vi "624WPI_CameraSend Images To PC Loop.vi"(4 "error in (no error) 2":errorcluster, 6 "port 2":u16=1180, 8 "CameraDevRef 2":T1, 9 "error in (no error)":errorcluster, 10 "port":u16=1180, 11 "CameraDevRef":T1) -> ()   [LabVIEW 2014]
doc: "This VI is used to send images to the dashboard using the second enet port on the 8 slot controller. This is provided for compatibility, but is higher overhead than using the Camera MJPG approach.\n\nThis software is licensed. Open the labview\\readme\\WPI Robotics Library Open Source License.txt file for more information."
uses:
  <vilib>/Rock Robotics/WPI/Camera/WPI_CameraDevRef.ctl
  <vilib>/Rock Robotics/SystemInterfaces/NetworkCommunication/NetComm_UsageReport_ResourceType.ctl
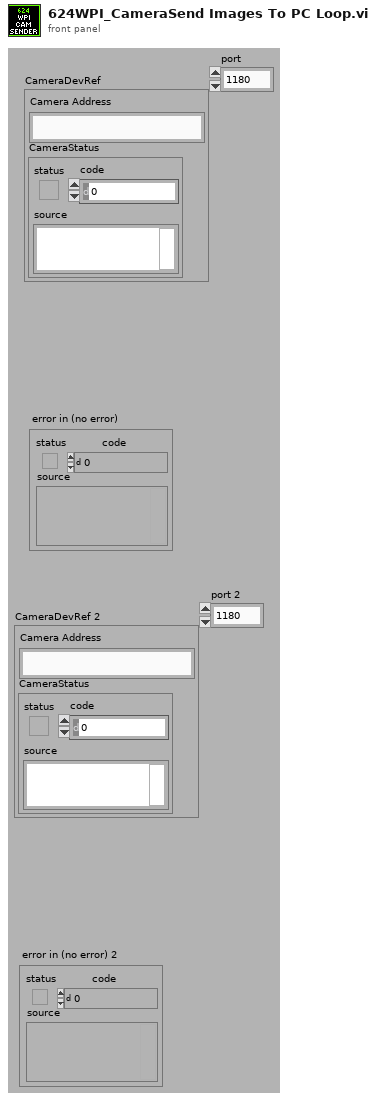
[diagram p1: front panel]
types:
  T1 = typedef "WPI_CameraDevRef.ctl" = cluster{"Camera Address":string, "CameraStatus":errorcluster}
  T2 = cluster{"fps":i32, "compression":i32, "compression 2":i32}
  T3 = typedef "NetComm_UsageReport_ResourceType.ctl" = enum8{"Controller", "Module", "Language", "CANPlugin", "Accelerometer", "ADXL345", "AnalogChannel", "AnalogTrigger", "AnalogTriggerOutput", "CANJaguar", "Compressor", "Counter", "Dashboard", "DigitalInput", "DigitalOutput", "DriverStationCIO", "DriverStationEIO", "DriverStationLCD", "Encoder", "GearTooth", "Gyro", "I2C", "Framework", "Jaguar", "Joystick", "Kinect", "KinectStick", "PIDController", "Preferences", "PWM", "Relay", "RobotDrive", "SerialPort", "Servo", "Solenoid", "SPI", "Task", "Ultrasonic", "Victor", "Button", "Command", "AxisCamera", "PCVideoServer", "SmartDashboard", "Talon", "HiTechnicColorSensor", "HiTechnicAccel", "HiTechnicCompass", "SRF08", "AnalogOutput", "Victor SP", "Talon SRX", "CAN Talon SRX"}
  T4 = enum16{"Update Mode", "Get Image", "Get Image Data"}
  T5 = typedef "Image Type" = u32
  T6 = typedef "IMAQ Image.ctl" = refnum<image>
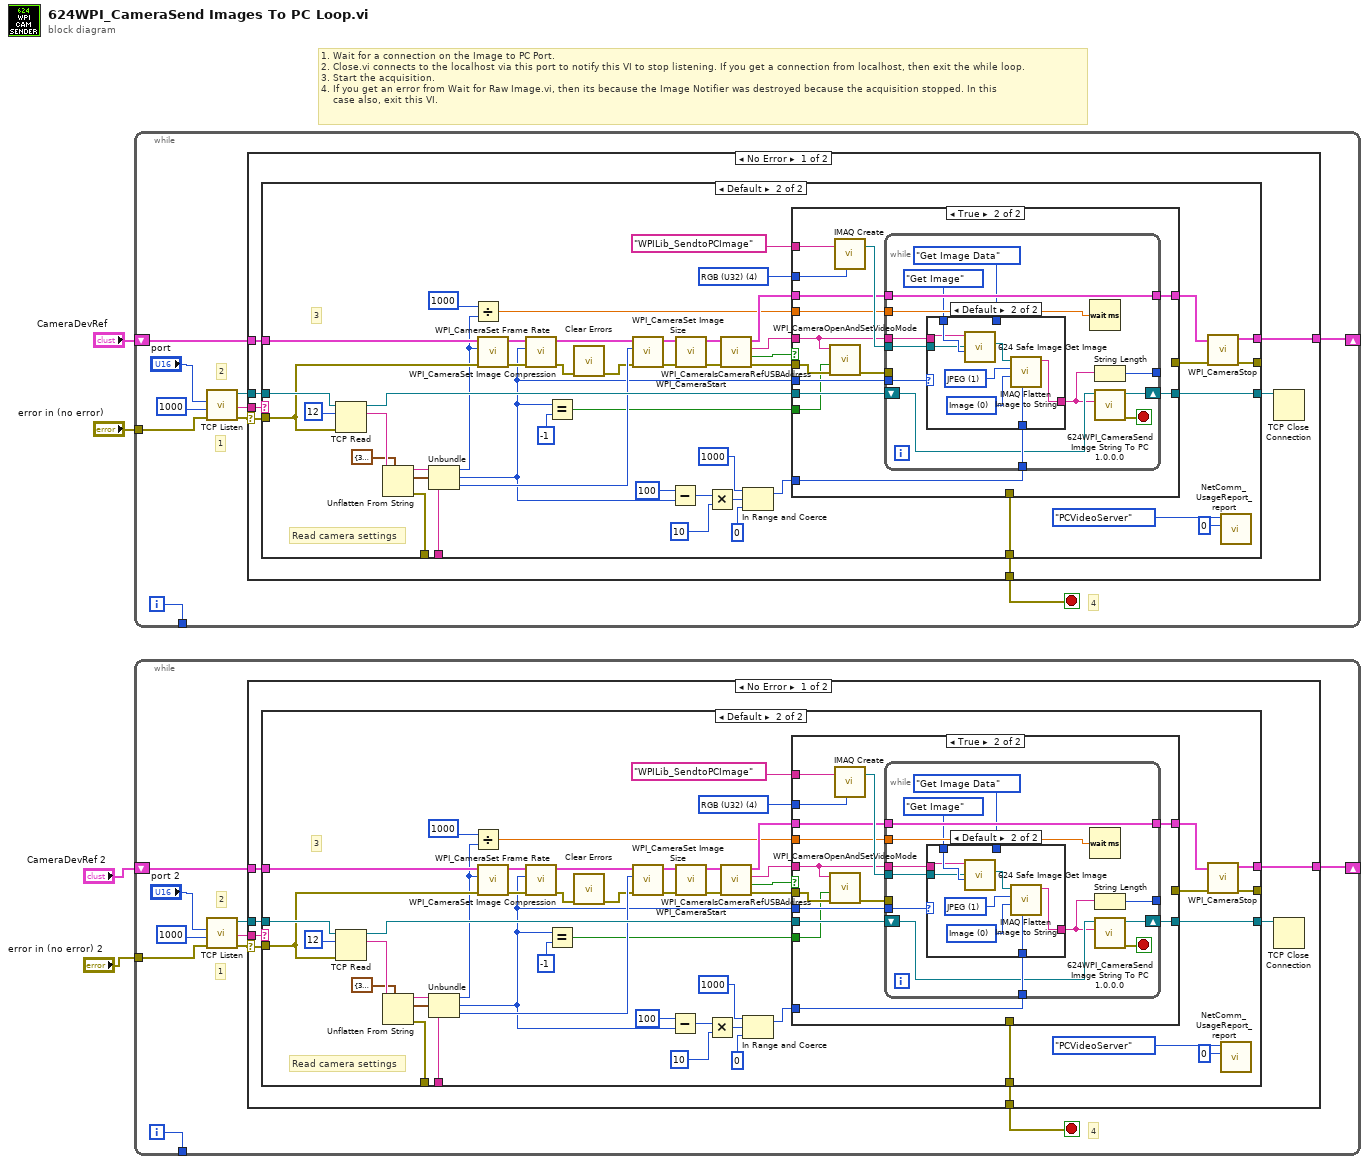
[diagram p0: block diagram]
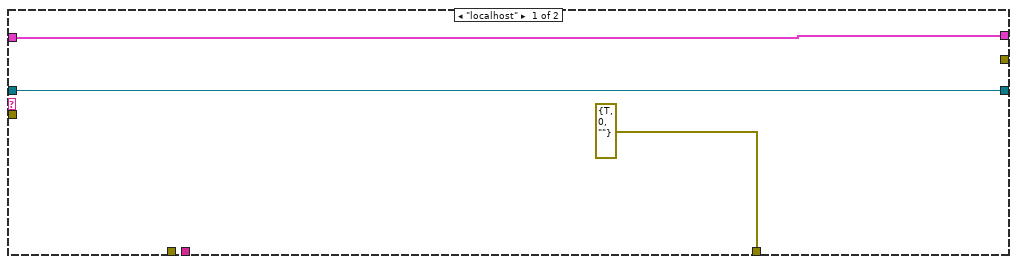
[diagram p2: hidden frame]
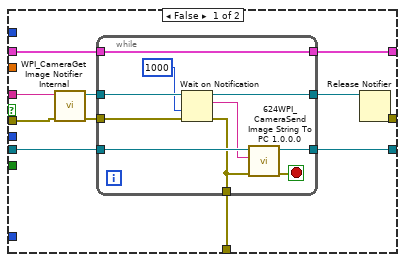
[diagram p3: hidden frame]
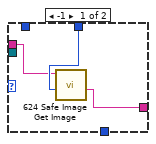
[diagram p4: hidden frame]
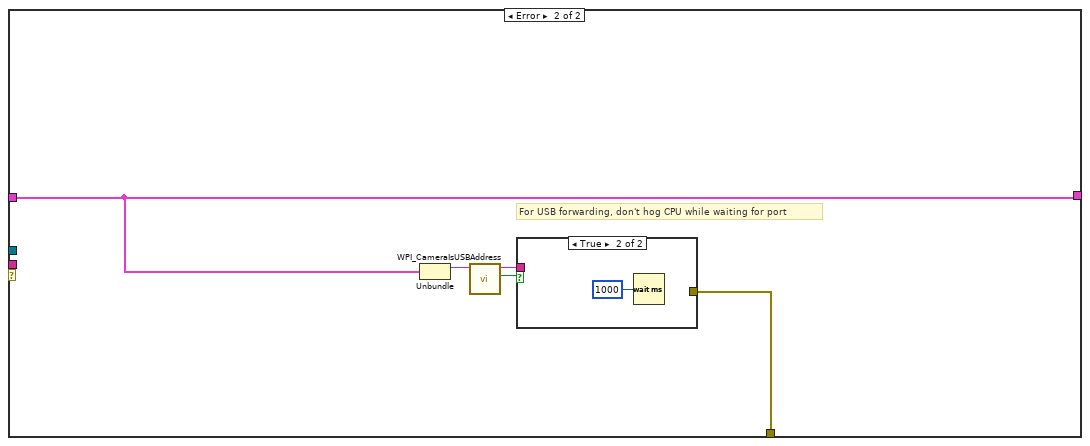
[diagram p5: hidden frame]
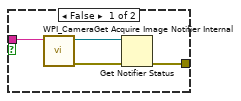
[diagram p6: hidden frame]
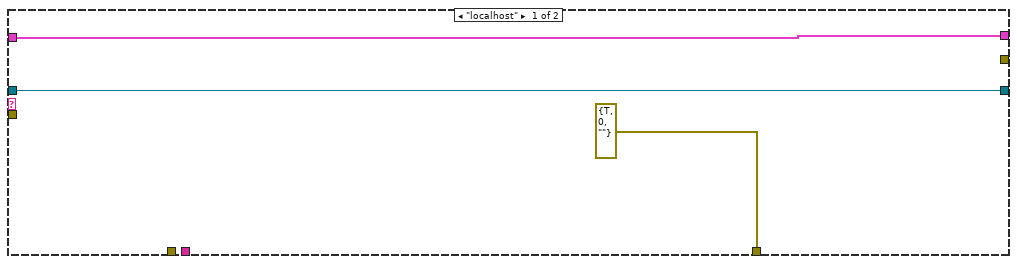
[diagram p7: hidden frame]
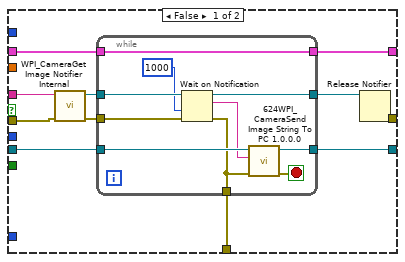
[diagram p8: hidden frame]
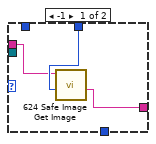
[diagram p9: hidden frame]
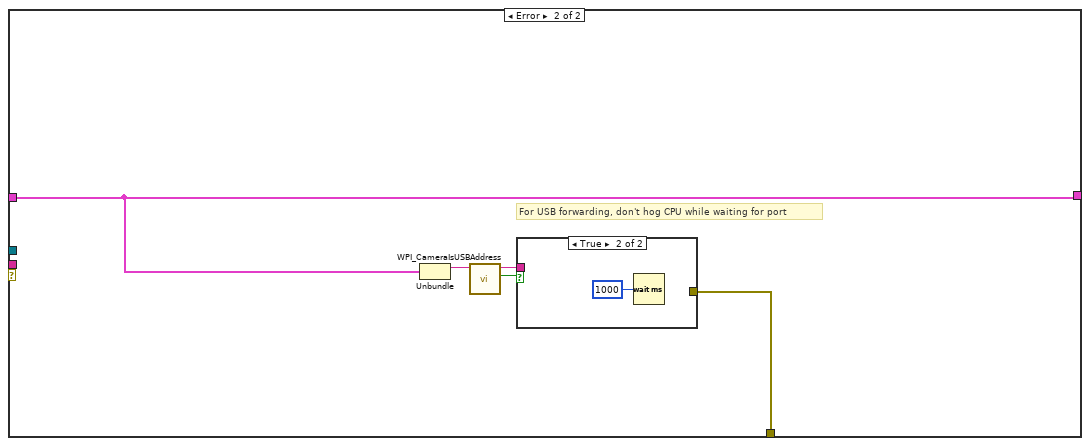
[diagram p10: hidden frame]
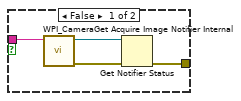
[diagram p11: hidden frame]
diagram:
  # "1. Wait for a connection on the Image to PC Port.\n2. Close.vi connects to the localhost via this port to notify this VI to stop listening. If you get a connection from localhost, then exit the while loop.\n3. Start the acquisition.\n4. If you get an error from Wait for Raw Image.vi, then its because the Image Notifier was destroyed because the acquisition stopped. In this\n    case also, exit this VI."
  n1 = while {
    tunnel: "error in (no error)" -> [w11]
    shift-right: [w14] -> _
    shift-left: "CameraDevRef" -> [w12]
    tunnel: [w6] -> _
    i -> [w6]
    stop <- w9 stop-if-true
    # "4"
    # "1"
    # "2"
    n2 = call <vilib>:"TCP Listen.vi"("error in (no error)"=w11, "timeout ms (wait forever: -1)"=u16 1000 ("port"), "port"="port") -> ("error out"=w8:errorcluster, "remote address"=w13:string, "connection ID"=w10:refnum<k5>)  [unwired: 1 in, 5 out]
    n3 = case shown="No Error" w8 {
      selector: w8 -> [w15 _]
      tunnel: [w21 w134] -> w14
      tunnel: w13 -> [w20 _]
      tunnel: w12 -> [w19 w134]
      tunnel: w10 -> [w18 _]
      tunnel: [w17 w135] -> w9
      frame No Error {
        n4 = case shown="Default" w20 {
          tunnel: [w24 w69] -> w21
          tunnel: w19 -> [w24 w51]
          tunnel: w15 -> [_ w47]
          tunnel: w18 -> [w22 w55]
          tunnel: [errorcluster {"status"=TRUE, "code"=0, "source"=""} ("error out 2") w71] -> w17
          tunnel: [w22 w70] -> w16
          tunnel: [_ w68] -> _
          tunnel: [_ w26] -> _
          tunnel: [_ w25] -> _
          frame "localhost" {
          }
          frame Default {
            w62 = T5 4 items=["Grayscale (U8)", "Grayscale (I16)", "Grayscale (SGL)", "Complex (CSG)", "RGB (U32)", "HSL (U32)", "RGB (U64)", "Grayscale (U16)"] ("Image Type")
            # "Read camera settings"
            # "3"
            n5 = TCP Read(connection ID=w55, bytes to read=12, error in (no error)=w47) -> (connection ID out=w54:refnum<k5>, data out=w52:string)  [unwired: 2 in, 1 out]
            n6 = Unflatten From String(type=T2 {"fps"=30, "compression"=32, "compression 2"=32} ("Camera Settings"), binary string=w52) -> (rest of the binary string=w25:string, value=w44:T2, error out=w26:errorcluster)  [unwired: 3 in]
            n7 = Unbundle(w44) -> ("fps"=w41:i32, "compression"=w30:i32, "compression 2"=w43:i32)
            n8 = Divide(x=u16 1000 ("port"), y=w41) -> (x/y=w40:dbl)
            n9 = call <vilib>:"WPI_CameraSet Frame Rate.vi"("error in (no error)"=w47, "Frame Rate (fps)"=w41, "CameraDevRef"=w51) -> ("error out"=w46:errorcluster, "CameraDevRef Out"=w50:T1)  [unwired: 7 in]
            n10 = call <vilib>:"WPI_CameraSet Image Compression.vi"("error in (no error)"=w46, "Compression"=w30, "CameraDevRef"=w50) -> ("error out"=w28:errorcluster, "CameraDevRef Out"=w49:T1)  [unwired: 7 in]
            n11 = Equal?(x=w30, y=-1) -> (x = y?=w29:bool)
            n12 = call <vilib>:"Clear Errors.vi"("error in (no error)"=w28) -> ("error out"=w27:errorcluster)  [unwired: 5 in, 1 out]
            n13 = call <vilib>:"WPI_CameraSet Image Size.vi"("error in (no error)"=w27, "Image Size"=w43, "CameraDevRef"=w49) -> ("error out"=w45:errorcluster, "CameraDevRef Out"=w48:T1)  [unwired: 7 in]
            n14 = Subtract(x=100, y=w30) -> (x-y=w35:i32)
            n15 = call <vilib>:"WPI_CameraStart.vi"("error in (no error)"=w45, "CameraDevRef"=w48) -> ("error out"=w59:errorcluster, "CameraDevRef Out"=w57:T1)  [unwired: 8 out]
            n16 = Multiply(x=w35, y=10) -> (x*y=w37:i32)
            n17 = call <vilib>:"WPI_CameraIsCameraRefUSBAddress.vi"("error in (no error)"=w59, "CameraDevRef"=w57) -> ("error out"=w58:errorcluster, "USB?"=w60:bool, "Camera Address Out"=w61:string, "CameraDevRef out"=w56:T1)  [unwired: 6 in]
            n18 = In Range and Coerce(upper limit=1000, x=w37, lower limit=0) -> (coerced(x)=w33:i32)  [unwired: 1 out]
            n19 = case shown="True" w60 {
              tunnel: w54 -> [w82 w106]
              tunnel: [w81 _] -> w71
              tunnel: [w80 w105] -> w70
              tunnel: w58 -> [w79 w96]
              tunnel: w61 -> [w77 w95]
              tunnel: [w76 w100] -> w67
              tunnel: w56 -> [w75 w101]
              tunnel: [w73 _] -> w66
              tunnel: "WPILib_SendtoPCImage" -> [_ w103]
              tunnel: w62 -> [_ w102]
              tunnel: w33 -> [_ w99]
              tunnel: w40 -> [_ w98]
              tunnel: w30 -> [_ w97]
              tunnel: w29 -> [_ w93]
              frame False {
                n20 = call <vilib>:"WPI_CameraGet Image Notifier Internal.vi"("error in (no error)"=w79, "Camera Address"=w77) -> ("error out"=w78:errorcluster, "Image Notifier"=w74:refnum<notifier>)  [unwired: 8 out]
                n21 = while {
                  tunnel: w78 -> [w88]
                  tunnel: w82 -> [w92]
                  tunnel: [w85] -> w81
                  tunnel: [w90] -> w80
                  tunnel: [w89] -> w76
                  tunnel: w75 -> [w89]
                  tunnel: w74 -> [w87]
                  tunnel: [w83] -> w72
                  stop <- w91 stop-if-true
                  n22 = Wait on Notification(notifier=w87, timeout in ms (-1)=1000 ("Timeout in ms (-1)"), error in (no error)=w88) -> (notifier out=w83:refnum<notifier>, notification=w86:string, error out=w85:errorcluster)  [unwired: 2 out]
                  n23 = call "624WPI_CameraSend Image String To PC 1.0.0.0.vi"("error in (no error)"=w85, "String"=w86, "TCP Connection ID"=w92) -> ("error out"=w91:errorcluster, "TCP Connection ID out"=w90:refnum<k5>)  [unwired: 7 out]
                }
                n24 = Release Notifier(notifier=w72) -> (error out=w73:errorcluster)  [unwired: 1 in, 3 out]
              }
              frame True {
                n25 = call <vilib>:"WPI_CameraOpenAndSetVideoMode.vi"("error in (no error)"=w96, "USB JPEG"=w93, "Camera Address Out"=w95) -> ("error out"=w94:errorcluster)  [unwired: 8 in]
                n26 = call "IMAQ Create"("Image Name"=w103, "Image Type"=w102) -> ("New Image"=w104:T6)  [unwired: 3 in, 1 out]
                n27 = while {
                  tunnel: w95 -> [w118]
                  shift-right: [w119] -> w105
                  shift-left: w106 -> [w112]
                  tunnel: w104 -> [w117]
                  tunnel: [w115] -> w100
                  tunnel: w101 -> [w115]
                  tunnel: w99 -> [w114]
                  tunnel: w98 -> [w113]
                  tunnel: [w110] -> _
                  tunnel: w97 -> [w109]
                  tunnel: w94 -> [_]
                  stop <- w116 stop-if-true
                  n28 = case shown="Default" w109 {
                    tunnel: [w121 w130] -> w111
                    tunnel: w118 -> [w120 w125]
                    tunnel: w117 -> [_ w124]
                    tunnel: w114 -> [_ w127]
                    tunnel: T4."Get Image Data" ("Operation") -> [w122 _]
                    tunnel: T4."Get Image" ("Operation") -> [_ w126]
                    frame -1 {
                      n29 = call "624 Safe Image Get Image.vi"("Operation"=w122, "Session In"=w120) -> ("Image Data String"=w121:string)  [unwired: 6 in, 3 out]
                    }
                    frame Default {
                      w128 = 0 items=["Image", "Image and Vision Info", "Reference to Image"] ("Type of Flatten (Image and Vision Info)")
                      w129 = 1 items=["None", "JPEG", "PACKED BINARY"] ("Compression (None)")
                      n30 = call "624 Safe Image Get Image.vi"("Operation"=w126, "Image In"=w124, "Session In"=w125) -> ("Image Out"=w123:T6)  [unwired: 5 in, 3 out]
                      n31 = call "IMAQ Flatten Image to String"("Quality (750)"=w127, "Type of Flatten (Image and Vision Info)"=w128, "Compression (None)"=w129, "Image"=w123) -> ("Data String"=w130:string)  [unwired: 6 in, 1 out]
                    }
                  }
                  n32 = Wait (ms)(milliseconds to wait=w113) -> ()  [unwired: 1 out]
                  n33 = String Length(string=w111) -> (length=w110:i32)
                  n34 = call "624WPI_CameraSend Image String To PC 1.0.0.0.vi"("String"=w111, "TCP Connection ID"=w112) -> ("error out"=w116:errorcluster, "TCP Connection ID out"=w119:refnum<k5>)  [unwired: 1 in, 7 out]
                }
              }
            }
            n35 = call <vilib>:"WPI_CameraStop.vi"("error in (no error)"=w66, "CameraDevRef"=w67) -> ("error out"=w68:errorcluster, "CameraDevRef Out"=w69:T1)  [unwired: 8 out]
            n36 = call <vilib>:"NetComm_UsageReport_report.vi"("Instance Number"=u8 0, "Resource Type"=NetComm_UsageReport_ResourceType."PCVideoServer") -> ()  [unwired: 10 in]
          }
        }
        n37 = TCP Close Connection(connection ID=w16) -> ()  [unwired: 1 in, 3 out]
      }
      frame Error {
        # "For USB forwarding, don't hog CPU while waiting for port"
        n38 = Unbundle(w134) -> ("Camera Address"=w133:string)  [unwired: 1 out]
        n39 = call <vilib>:"WPI_CameraIsUSBAddress.vi"("Camera Address In"=w133) -> ("USB?"=w131:bool, "Camera Address Out"=w132:string)  [unwired: 8 in, 1 out]
        n40 = case shown="True" w131 {
          tunnel: [w139 _] -> w135
          tunnel: w132 -> [w136 _]
          frame False {
            n41 = call <vilib>:"WPI_CameraGet Acquire Image Notifier Internal.vi"("Camera Address"=w136) -> ("error out"=w137:errorcluster, "Acquire Image Notifier"=w138:refnum<notifier>)  [unwired: 1 in, 8 out]
            n42 = Get Notifier Status(notifier=w138, error in (no error)=w137) -> (error out=w139:errorcluster)  [unwired: 4 out]
          }
          frame True {
            n43 = Wait (ms)(milliseconds to wait=u32 1000) -> ()  [unwired: 1 out]
          }
        }
      }
    }
  }
  n44 = while {
    tunnel: "error in (no error) 2" -> [w147]
    shift-right: [w150] -> _
    shift-left: "CameraDevRef 2" -> [w148]
    tunnel: [w142] -> _
    i -> [w142]
    stop <- w145 stop-if-true
    # "4"
    # "1"
    # "2"
    n45 = call <vilib>:"TCP Listen.vi"("error in (no error)"=w147, "timeout ms (wait forever: -1)"=u16 1000 ("port"), "port"="port 2") -> ("error out"=w144:errorcluster, "remote address"=w149:string, "connection ID"=w146:refnum<k5>)  [unwired: 1 in, 5 out]
    n46 = case shown="No Error" w144 {
      selector: w144 -> [w151 _]
      tunnel: [w157 w270] -> w150
      tunnel: w149 -> [w156 _]
      tunnel: w148 -> [w155 w270]
      tunnel: w146 -> [w154 _]
      tunnel: [w153 w271] -> w145
      frame No Error {
        n47 = case shown="Default" w156 {
          tunnel: [w160 w205] -> w157
          tunnel: w155 -> [w160 w187]
          tunnel: w151 -> [_ w183]
          tunnel: w154 -> [w158 w191]
          tunnel: [errorcluster {"status"=TRUE, "code"=0, "source"=""} ("error out 2") w207] -> w153
          tunnel: [w158 w206] -> w152
          tunnel: [_ w204] -> _
          tunnel: [_ w162] -> _
          tunnel: [_ w161] -> _
          frame "localhost" {
          }
          frame Default {
            w198 = T5 4 items=["Grayscale (U8)", "Grayscale (I16)", "Grayscale (SGL)", "Complex (CSG)", "RGB (U32)", "HSL (U32)", "RGB (U64)", "Grayscale (U16)"] ("Image Type")
            # "Read camera settings"
            # "3"
            n48 = TCP Read(connection ID=w191, bytes to read=12, error in (no error)=w183) -> (connection ID out=w190:refnum<k5>, data out=w188:string)  [unwired: 2 in, 1 out]
            n49 = Unflatten From String(type=T2 {"fps"=30, "compression"=32, "compression 2"=32} ("Camera Settings"), binary string=w188) -> (rest of the binary string=w161:string, value=w180:T2, error out=w162:errorcluster)  [unwired: 3 in]
            n50 = Unbundle(w180) -> ("fps"=w177:i32, "compression"=w166:i32, "compression 2"=w179:i32)
            n51 = Divide(x=u16 1000 ("port"), y=w177) -> (x/y=w176:dbl)
            n52 = call <vilib>:"WPI_CameraSet Frame Rate.vi"("error in (no error)"=w183, "Frame Rate (fps)"=w177, "CameraDevRef"=w187) -> ("error out"=w182:errorcluster, "CameraDevRef Out"=w186:T1)  [unwired: 7 in]
            n53 = call <vilib>:"WPI_CameraSet Image Compression.vi"("error in (no error)"=w182, "Compression"=w166, "CameraDevRef"=w186) -> ("error out"=w164:errorcluster, "CameraDevRef Out"=w185:T1)  [unwired: 7 in]
            n54 = Equal?(x=w166, y=-1) -> (x = y?=w165:bool)
            n55 = call <vilib>:"Clear Errors.vi"("error in (no error)"=w164) -> ("error out"=w163:errorcluster)  [unwired: 5 in, 1 out]
            n56 = call <vilib>:"WPI_CameraSet Image Size.vi"("error in (no error)"=w163, "Image Size"=w179, "CameraDevRef"=w185) -> ("error out"=w181:errorcluster, "CameraDevRef Out"=w184:T1)  [unwired: 7 in]
            n57 = Subtract(x=100, y=w166) -> (x-y=w171:i32)
            n58 = call <vilib>:"WPI_CameraStart.vi"("error in (no error)"=w181, "CameraDevRef"=w184) -> ("error out"=w195:errorcluster, "CameraDevRef Out"=w193:T1)  [unwired: 8 out]
            n59 = Multiply(x=w171, y=10) -> (x*y=w173:i32)
            n60 = call <vilib>:"WPI_CameraIsCameraRefUSBAddress.vi"("error in (no error)"=w195, "CameraDevRef"=w193) -> ("error out"=w194:errorcluster, "USB?"=w196:bool, "Camera Address Out"=w197:string, "CameraDevRef out"=w192:T1)  [unwired: 6 in]
            n61 = In Range and Coerce(upper limit=1000, x=w173, lower limit=0) -> (coerced(x)=w169:i32)  [unwired: 1 out]
            n62 = case shown="True" w196 {
              tunnel: w190 -> [w218 w242]
              tunnel: [w217 _] -> w207
              tunnel: [w216 w241] -> w206
              tunnel: w194 -> [w215 w232]
              tunnel: w197 -> [w213 w231]
              tunnel: [w212 w236] -> w203
              tunnel: w192 -> [w211 w237]
              tunnel: [w209 _] -> w202
              tunnel: "WPILib_SendtoPCImage" -> [_ w239]
              tunnel: w198 -> [_ w238]
              tunnel: w169 -> [_ w235]
              tunnel: w176 -> [_ w234]
              tunnel: w166 -> [_ w233]
              tunnel: w165 -> [_ w229]
              frame False {
                n63 = call <vilib>:"WPI_CameraGet Image Notifier Internal.vi"("error in (no error)"=w215, "Camera Address"=w213) -> ("error out"=w214:errorcluster, "Image Notifier"=w210:refnum<notifier>)  [unwired: 8 out]
                n64 = while {
                  tunnel: w214 -> [w224]
                  tunnel: w218 -> [w228]
                  tunnel: [w221] -> w217
                  tunnel: [w226] -> w216
                  tunnel: [w225] -> w212
                  tunnel: w211 -> [w225]
                  tunnel: w210 -> [w223]
                  tunnel: [w219] -> w208
                  stop <- w227 stop-if-true
                  n65 = Wait on Notification(notifier=w223, timeout in ms (-1)=1000 ("Timeout in ms (-1)"), error in (no error)=w224) -> (notifier out=w219:refnum<notifier>, notification=w222:string, error out=w221:errorcluster)  [unwired: 2 out]
                  n66 = call "624WPI_CameraSend Image String To PC 1.0.0.0.vi"("error in (no error)"=w221, "String"=w222, "TCP Connection ID"=w228) -> ("error out"=w227:errorcluster, "TCP Connection ID out"=w226:refnum<k5>)  [unwired: 7 out]
                }
                n67 = Release Notifier(notifier=w208) -> (error out=w209:errorcluster)  [unwired: 1 in, 3 out]
              }
              frame True {
                n68 = call <vilib>:"WPI_CameraOpenAndSetVideoMode.vi"("error in (no error)"=w232, "USB JPEG"=w229, "Camera Address Out"=w231) -> ("error out"=w230:errorcluster)  [unwired: 8 in]
                n69 = call "IMAQ Create"("Image Name"=w239, "Image Type"=w238) -> ("New Image"=w240:T6)  [unwired: 3 in, 1 out]
                n70 = while {
                  tunnel: w231 -> [w254]
                  shift-right: [w255] -> w241
                  shift-left: w242 -> [w248]
                  tunnel: w240 -> [w253]
                  tunnel: [w251] -> w236
                  tunnel: w237 -> [w251]
                  tunnel: w235 -> [w250]
                  tunnel: w234 -> [w249]
                  tunnel: [w246] -> _
                  tunnel: w233 -> [w245]
                  tunnel: w230 -> [_]
                  stop <- w252 stop-if-true
                  n71 = case shown="Default" w245 {
                    tunnel: [w257 w266] -> w247
                    tunnel: w254 -> [w256 w261]
                    tunnel: w253 -> [_ w260]
                    tunnel: w250 -> [_ w263]
                    tunnel: T4."Get Image Data" ("Operation") -> [w258 _]
                    tunnel: T4."Get Image" ("Operation") -> [_ w262]
                    frame -1 {
                      n72 = call "624 Safe Image Get Image.vi"("Operation"=w258, "Session In"=w256) -> ("Image Data String"=w257:string)  [unwired: 6 in, 3 out]
                    }
                    frame Default {
                      w264 = 0 items=["Image", "Image and Vision Info", "Reference to Image"] ("Type of Flatten (Image and Vision Info)")
                      w265 = 1 items=["None", "JPEG", "PACKED BINARY"] ("Compression (None)")
                      n73 = call "624 Safe Image Get Image.vi"("Operation"=w262, "Image In"=w260, "Session In"=w261) -> ("Image Out"=w259:T6)  [unwired: 5 in, 3 out]
                      n74 = call "IMAQ Flatten Image to String"("Quality (750)"=w263, "Type of Flatten (Image and Vision Info)"=w264, "Compression (None)"=w265, "Image"=w259) -> ("Data String"=w266:string)  [unwired: 6 in, 1 out]
                    }
                  }
                  n75 = Wait (ms)(milliseconds to wait=w249) -> ()  [unwired: 1 out]
                  n76 = String Length(string=w247) -> (length=w246:i32)
                  n77 = call "624WPI_CameraSend Image String To PC 1.0.0.0.vi"("String"=w247, "TCP Connection ID"=w248) -> ("error out"=w252:errorcluster, "TCP Connection ID out"=w255:refnum<k5>)  [unwired: 1 in, 7 out]
                }
              }
            }
            n78 = call <vilib>:"WPI_CameraStop.vi"("error in (no error)"=w202, "CameraDevRef"=w203) -> ("error out"=w204:errorcluster, "CameraDevRef Out"=w205:T1)  [unwired: 8 out]
            n79 = call <vilib>:"NetComm_UsageReport_report.vi"("Instance Number"=u8 0, "Resource Type"=NetComm_UsageReport_ResourceType."PCVideoServer") -> ()  [unwired: 10 in]
          }
        }
        n80 = TCP Close Connection(connection ID=w152) -> ()  [unwired: 1 in, 3 out]
      }
      frame Error {
        # "For USB forwarding, don't hog CPU while waiting for port"
        n81 = Unbundle(w270) -> ("Camera Address"=w269:string)  [unwired: 1 out]
        n82 = call <vilib>:"WPI_CameraIsUSBAddress.vi"("Camera Address In"=w269) -> ("USB?"=w267:bool, "Camera Address Out"=w268:string)  [unwired: 8 in, 1 out]
        n83 = case shown="True" w267 {
          tunnel: [w275 _] -> w271
          tunnel: w268 -> [w272 _]
          frame False {
            n84 = call <vilib>:"WPI_CameraGet Acquire Image Notifier Internal.vi"("Camera Address"=w272) -> ("error out"=w273:errorcluster, "Acquire Image Notifier"=w274:refnum<notifier>)  [unwired: 1 in, 8 out]
            n85 = Get Notifier Status(notifier=w274, error in (no error)=w273) -> (error out=w275:errorcluster)  [unwired: 4 out]
          }
          frame True {
            n86 = Wait (ms)(milliseconds to wait=u32 1000) -> ()  [unwired: 1 out]
          }
        }
      }
    }
  }
